vi "[Timestamped File] High-Level Write to Text File.vi"() -> ()   [LabVIEW 2019]
uses:
  <vilib>/DAQmx/read.llb/DAQmx Read (Analog 2D DBL NChan NSamp).vi
  <vilib>/DAQmx/create/channels.llb/DAQmx Create Channel (AI-Voltage-Basic).vi
  <vilib>/DAQmx/configure/timing.llb/DAQmx Timing (Sample Clock).vi
  <vilib>/DAQmx/miscellaneous.llb/DAQmx Fill In Error Info.vi
  <vilib>/Utility/file.llb/Write Delimited Spreadsheet (string).vi
  <vilib>/Utility/file.llb/Write Delimited Spreadsheet (DBL).vi
  <resource>/objmgr/daqmx.rc
panel:
  in  "maximum value":dbl=5.0
  in  "minimum value":dbl=-5.0
  out "Waveform Graph":dbl[][](graph)
  in  "Number of Samples":i32=100
  in  "Desired Sample Rate (Hz)":dbl=1000.0
  in  "Physical Channels":tag="PCI-6221/ai0:3"
  out "Actual Sample Rate (Hz)":dbl
  # "Measurement Range"
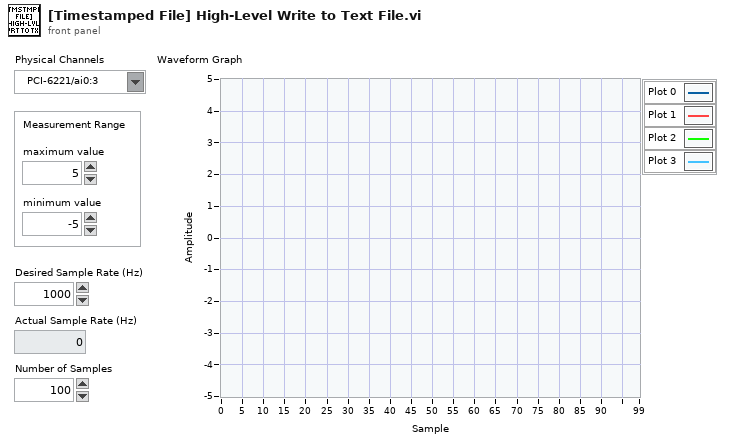
[diagram p1: front panel]
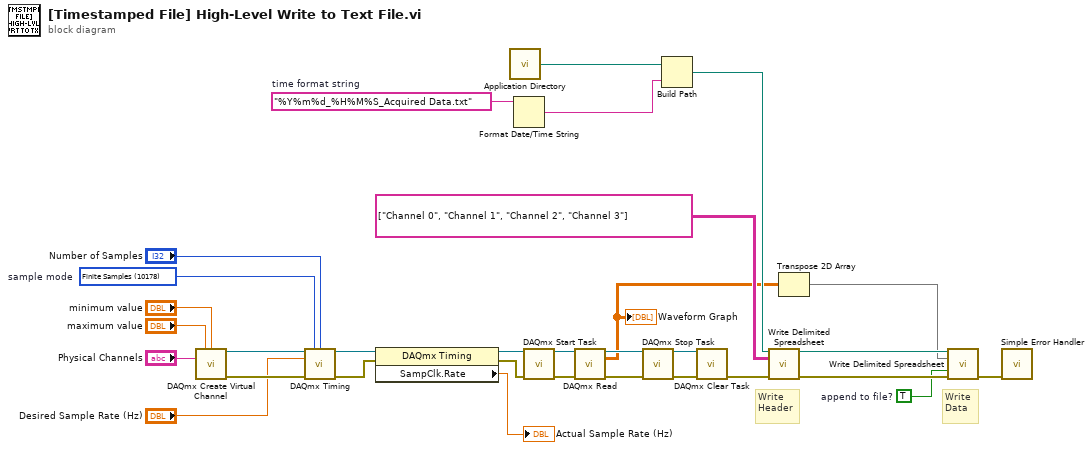
[diagram p0: block diagram]
diagram:
  w9 = TRUE  # append to file?
  w28 = 10178 items=["Finite Samples"=10178, "Continuous Samples"=10123, "Hardware Timed Single Point"=12522]  # sample mode
  w31 = "%Y%m%d_%H%M%S_Acquired Data.txt"  # time format string
  # "Write Data"
  # "Write Header"
  n1 = call-poly <vilib>:"DAQmx Create Virtual Channel.vi"("maximum value"="maximum value", "minimum value"="minimum value", "physical channels"="Physical Channels") -> ("task out"=w27:refnum<k21>, "error out"=w26:errorcluster)  [unwired: 11 in]
  n2 = call-poly <vilib>:"DAQmx Timing.vi"("task/channels in"=w27, "sample mode"=w28, "samples per channel"="Number of Samples", "rate"="Desired Sample Rate (Hz)", "error in"=w26) -> ("task out"=w25:refnum<k21>, "error out"=w24:errorcluster)  [unwired: 9 in]
  n3 = property class="DAQmx Timing"(reference=w25, error in=w24) -> (reference out=w23:refnum<k21>, error out=w22:errorcluster, "SampClk.Rate"=→"Actual Sample Rate (Hz)":dbl)
  n4 = call <vilib>:"Application Directory.vi"() -> ("Application Directory"=w30:path)
  n5 = Format Date/Time String(time format string (%c)=w31) -> (date/time string=w29:string)  [unwired: 2 in]
  n6 = call <vilib>:"DAQmx Start Task.vi"("task/channels in"=w23, "error in"=w22) -> ("task out"=w21:refnum<k21>, "error out"=w20:errorcluster)  [unwired: 12 in]
  n7 = call-poly <vilib>:"DAQmx Read.vi"("task/channels in"=w21, "error in"=w20) -> ("task out"=w19:refnum<k21>, "data"=w2:dbl[][], "error out"=w18:errorcluster)  [unwired: 11 in]
  "Waveform Graph" <- w2
  n8 = call <vilib>:"DAQmx Stop Task.vi"("task/channels in"=w19, "error in"=w18) -> ("task out"=w17:refnum<k21>, "error out"=w16:errorcluster)  [unwired: 12 in]
  n9 = Build Path(base path=w30, name or relative path=w29) -> (appended path=w13:path)
  n10 = call <vilib>:"DAQmx Clear Task.vi"("task in"=w17, "error in"=w16) -> ("error out"=w15:errorcluster)  [unwired: 13 in]
  n11 = call-poly <vilib>:"Write Delimited Spreadsheet.vi"("file path (dialog if empty)"=w13, "2D data"=string[][] [["Channel 0", "Channel 1", "Channel 2", "Channel 3"]], "error in (no error)"=w15) -> ("new file path (Not A Path if cancelled)"=w12:path, "error out"=w10:errorcluster)  [unwired: 11 in]
  n12 = Transpose 2D Array(2D array=w2) -> (transposed array=w11:dbl[][])
  n13 = call-poly <vilib>:"Write Delimited Spreadsheet.vi"("file path (dialog if empty)"=w12, "2D data"=w11, "append to file? (new file:F)"=w9, "error in (no error)"=w10) -> ("error out"=w8:errorcluster)  [unwired: 10 in, 1 out]
  n14 = call <vilib>:"Simple Error Handler.vi"("error in (no error)"=w8) -> ()  [unwired: 4 in, 5 out]
